vi "Create and Add Tasks.vi"(7 "Tasks <JSON>":string, 8 "error in (no error)":errorcluster, 11 "Study Base in":refnum<class "Study Base.lvclass">) -> (0 "error out":errorcluster, 3 "Study Base out":refnum<class "Study Base.lvclass">)   [LabVIEW 2023, in "HAL GOOP4.lvlib" / "Study Base.lvclass"]
uses:
  Study Base.lvclass
  Task Base/Task Base.lvclass
  Task Base/Task Base.lvclass/Task Base.ctl
  Study Base.lvclass/Study Base.ctl
  <vilib>/Utility/miscctls.llb/LVMapReplaceAction.ctl
  b874e428-42f4-4ebe-8b0a-882075bdcbe6.vi
  <vilib>/JDP Science/JSONtext/Find Item.vi
  <vilib>/JDP Science/JSONtext/Next JSON Value.vi
  <vilib>/JDP Science/JSONtext/String Subset.vi
  <vilib>/JDP Science/JSONtext/Parsing/Advance past next JSON Value (inlined COPY).vi
  <vilib>/JDP Science/JSONtext/Parsing/Advance past whitespace.vi
  <vilib>/JDP Science/JSONtext/Parsing/Advance past String.vi
  <vilib>/JDP Science/JSONtext/Parsing/Advance past Number.vi
  <vilib>/JDP Science/JSONtext/Parsing/Advance past Line Ending.vi
  <vilib>/JDP Science/JSONtext/Parsing/Parse Full Path or Item Name.vi
  <vilib>/JDP Science/JSONtext/Parsing/Advance past Array.vi
  <vilib>/JDP Science/JSONtext/Parsing/Advance past Object.vi
  <vilib>/JDP Science/JSONtext/support/Error Cluster From Code.vi
  <vilib>/JDP Science/JSONtext/Offset/Find Item Locations by Path.vi
  <vilib>/JDP Science/JSONtext/JSON text to Variant.vi
  <vilib>/Utility/error.llb/Error Cluster From Error Code.vi
  <vilib>/JDP Science/JSONtext/LVClass Serializer/JSONtext LVClass Serializer.lvclass
  <vilib>/ErrorRing/Error Ring.xnode
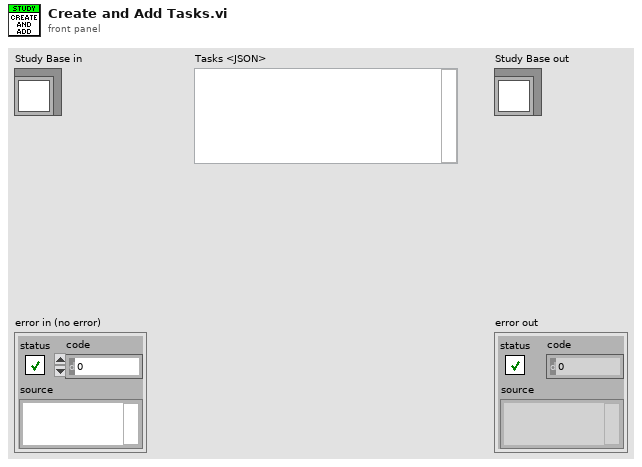
[diagram p1: front panel]
types:
  T1 = typedef "LVMapReplaceAction.ctl" = enum32{"Modify Entry only if found", "Add or Modify Entry", "Delete Entry"}
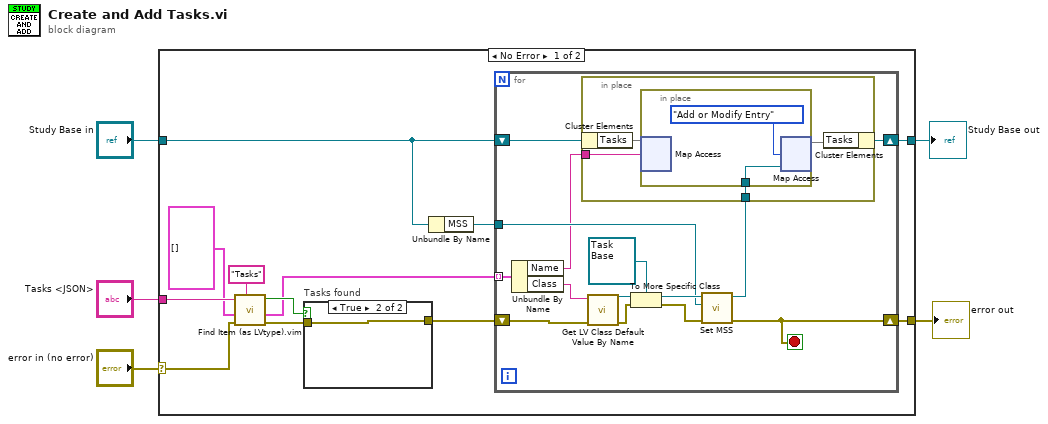
[diagram p0: block diagram]
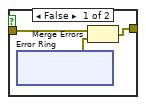
[diagram p2: hidden frame]
diagram:
  n1 = case shown="No Error" "error in (no error)" {
    selector: "error in (no error)" -> [w15 w48]
    tunnel: [w9 w48] -> w4
    tunnel: [w8 w47] -> w2
    tunnel: "Study Base in" -> [w7 w47]
    tunnel: "Tasks <JSON>" -> [w17 _]
    frame No Error {
      n2 = call "Find Item (as LVtype).vim"("$Path or Item Name"="Tasks", "error in (no error)"=w15, "Data Type and Default Value"=cluster{"Name":string, "Class":string}[] [] ("Tasks"), "JSON"=w17) -> ("error out"=w12:errorcluster, "Data"=w11:cluster{"Name":string, "Class":string}[], "Found"=w13:bool)  [unwired: 4 in, 1 out]
      n3 = case "Tasks found" shown="True" w13 {
        tunnel: w12 -> [w40 w46]
        tunnel: [w39 w46] -> w10
        frame False {
          n4 = xnode "Error Ring"() -> ("error out"=w38:errorcluster)
          n5 = Merge Errors(w40, w38) -> (w39:errorcluster)
        }
        frame True {
        }
      }
      n6 = Unbundle By Name(w7) -> ("MSS"=w6:refnum<class "Measure and Stimulus Subsystems.lvclass">)
      n7 = for {
        tunnel: w11 -> [w28] mode=indexing
        shift-right: [w22] -> w9
        shift-left: w10 -> [w27]
        tunnel: w6 -> [w21]
        shift-right: [w18] -> w8
        shift-left: w7 -> [w25]
        stop <- w22 stop-if-true
        n8 = Unbundle By Name(w28) -> ("Name"=w19:string, "Class"=w26:string)
        n9 = call <vilib>:"Get LV Class Default Value By Name.vi"("error in (no error)"=w27, "class name"=w26) -> ("error out"=w31:errorcluster, "object"=w30:refnum<class>)  [unwired: 8 in]
        n10 = To More Specific Class(target class=refnum<class "Task Base.lvclass"> refnum ("HAL GOOP4.lvlib:Task Base.lvclass"), reference=w30, error in=w31) -> (specific class reference=w24:refnum<class "Task Base.lvclass">, error out=w23:errorcluster)
        n11 = call "Set MSS.vi"("error in (no error)"=w23, "MSS"=w21, "Task Base in"=w24) -> ("error out"=w22:errorcluster, "Task Base out"=w20:refnum<class "Task Base.lvclass">)  [unwired: 7 in]
        n12 = in-place {
          in-place-border: w20 -> [w34]
          in-place-border: w19 -> [w33]
          n13 = in-place-cluster #1(w25) -> ("Tasks"=w35:map{string, refnum<class "Task Base.lvclass">})
          n14 = in-place {
            in-place-border: w34 -> [w37]
            n15 = in-place-map #2(w35, w33) -> ()  [unwired: 1 in, 2 out]
            n16 = in-place-map #2(w37, LVMapReplaceAction."Add or Modify Entry" ("action")) -> (w32:map{string, refnum<class "Task Base.lvclass">})  [unwired: 2 out]
          }
          n17 = in-place-cluster #1("Tasks"=w32) -> (w18:refnum<class "Study Base.lvclass">)
        }
      }
    }
    frame Error {
    }
  }
  "error out" <- w4
  "Study Base out" <- w2
